vi "Data File Processing UI Add Messages.vi"(8 "error in":errorcluster, 10 "messages":T1[](array[typedef]), 11 "msg queue in":refnum<queue>) -> (0 "error out":errorcluster, 3 "msg queue out":refnum<queue>)   [LabVIEW 2012]
uses:
  Data File Processing UI Message Define.ctl
  Data File Processing UI Message Type Define.ctl
panel:
  in  "time out":i32=-1
  # "Input Data"
  # "Local Data"
  # "Output Data"
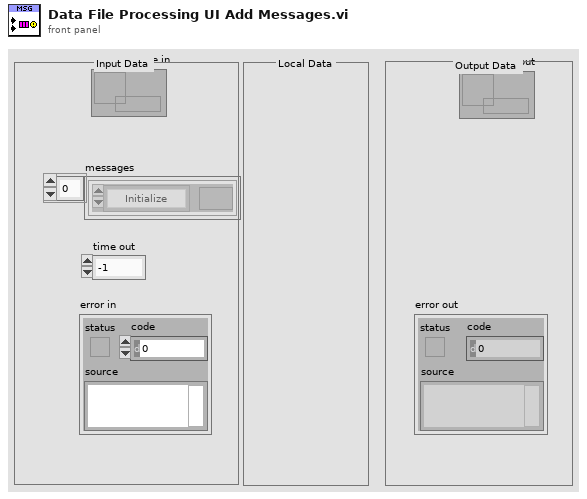
[diagram p1: front panel]
types:
  T1 = typedef "Data File Processing UI Message Define.ctl" = cluster{"data":variant, "type":T2}
  T2 = typedef "Data File Processing UI Message Type Define.ctl" = enum32{"Initialize", "SleepThread", "ErrorHandler", "NoEvent", "PreExit", "Exit", "----Action----", "OpenFile", "ReadAllCompute", "SaveFile", "RedrawGraph", "SelectChannel"}
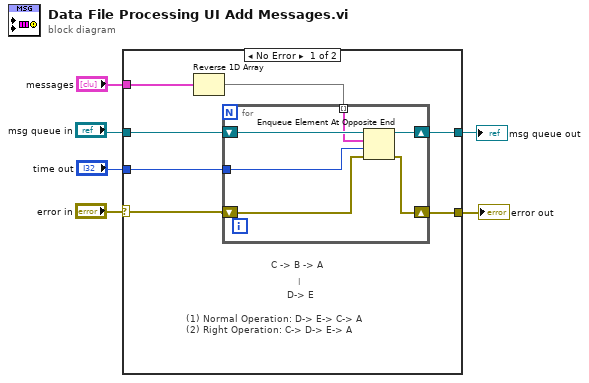
[diagram p0: block diagram]
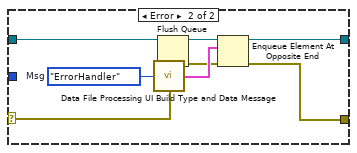
[diagram p2: hidden frame]
diagram:
  n1 = case shown="No Error" "error in" {
    selector: "error in" -> [w7 w21]
    tunnel: "messages" -> [w13 _]
    tunnel: "time out" -> [w12 _]
    tunnel: [w11 w26] -> w4
    tunnel: "msg queue in" -> [w9 w27]
    tunnel: [w8 w24] -> w2
    frame No Error {
      # "(1) Normal Operation: D-> E-> C-> A\n(2) Right Operation: C-> D-> E-> A"
      # "D-> E"
      # "|"
      # "C -> B -> A"
      n2 = Reverse 1D Array(array=w13) -> (reversed array=w10:T1[])
      n3 = for {
        tunnel: w10 -> [w14] mode=indexing
        shift-right: [w18] -> w8
        shift-left: w9 -> [w19]
        tunnel: w12 -> [w17]
        shift-right: [w15] -> w11
        shift-left: w7 -> [w16]
        n4 = Enqueue Element At Opposite End(queue=w19, element=w14, timeout in ms (-1)=w17, error in (no error)=w16) -> (queue out=w18:refnum<queue>, error out=w15:errorcluster)  [unwired: 1 out]
      }
    }
    frame Error {
      w23 = Data_File_Processing_UI_Message_Type_Define."ErrorHandler"  # Msg
      n5 = call "Data File Processing UI Build Type and Data Message.vi"("type"=w23, "data"=w21) -> ("msg out"=w25:T1)  [unwired: 13 out]
      n6 = Flush Queue(queue=w27) -> (queue out=w22:refnum<queue>, error out=w20:errorcluster)  [unwired: 1 in, 1 out]
      n7 = Enqueue Element At Opposite End(queue=w22, element=w25, error in (no error)=w20) -> (queue out=w24:refnum<queue>, error out=w26:errorcluster)  [unwired: 1 in, 1 out]
    }
  }
  "error out" <- w4
  "msg queue out" <- w2
